vi "config serial port.vi"(8 "error in (no error)":errorcluster) -> (0 "error out":errorcluster, 3 "reference out":refnum<visa-resource-name>)   [LabVIEW 2020]
uses:
  Ardunio Type.ctl
  <vilib>/Instr/_visa.llb/VISA Find Search Mode.ctl
  <vilib>/Instr/_visa.llb/VISA Configure Serial Port (Instr).vi
panel:
  out "find list":string[](array[string])
  out "Array":string[](array[string])
  out "Arduino Found":bool
  in  "Arduino type":T1
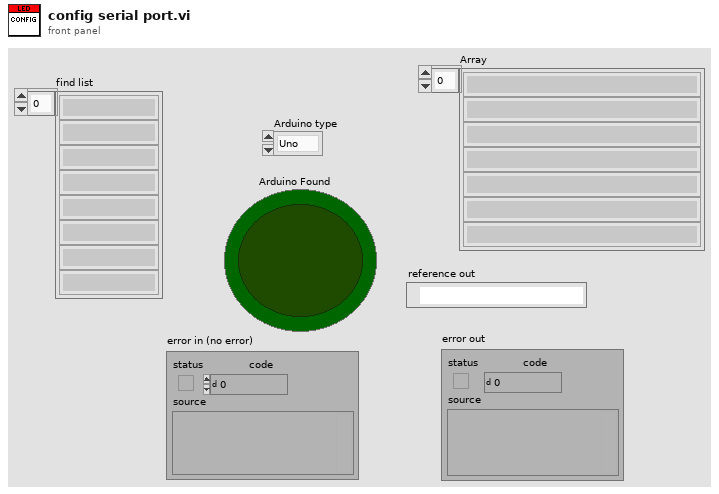
[diagram p1: front panel]
types:
  T1 = typedef "Ardunio Type.ctl" = enum16{"Uno", "Nano", "Micro"}
  T2 = typedef "VISA Find Search Mode.ctl" = u32
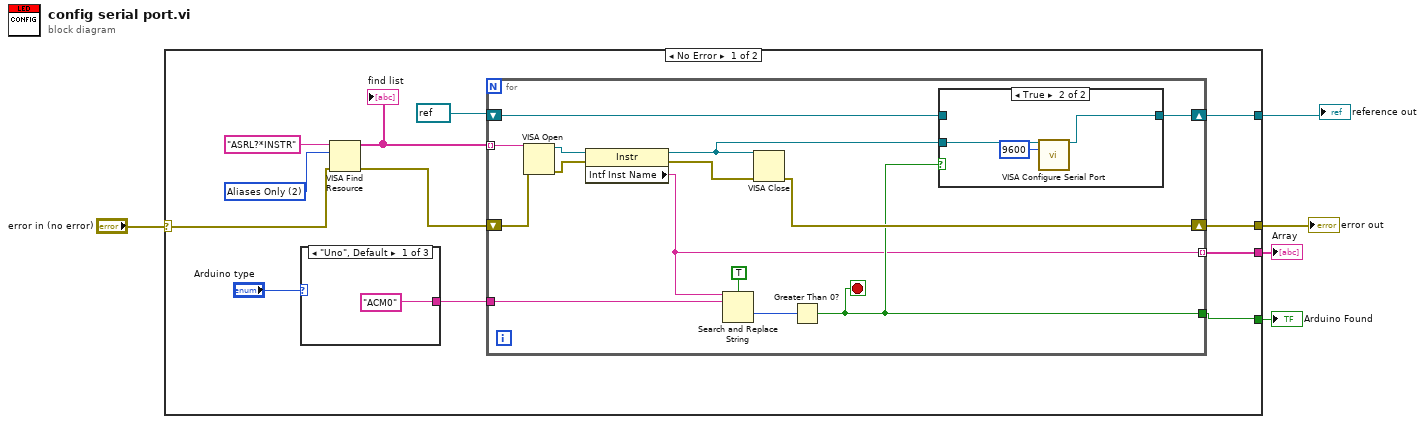
[diagram p0: block diagram]
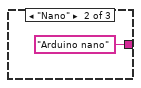
[diagram p2: hidden frame]
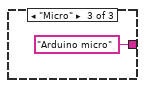
[diagram p3: hidden frame]
diagram:
  n1 = case shown="No Error" "error in (no error)" {
    selector: "error in (no error)" -> [w13 w39]
    tunnel: [w9 w39] -> w4
    tunnel: [w8 _] -> w3
    tunnel: [w7 _] -> w1
    tunnel: [w6 _] -> w2
    frame No Error {
      w16 = T2 2 items=["Canonical Names Only"=0, "Aliases Only"=2, "Include Matching Aliases"=3, "Include All Aliases"=4] ("Search Mode")
      n2 = case shown="\"Uno\", Default" "Arduino type" {
        tunnel: ["ACM0" ("search string") "Arduino nano" ("search string") "Arduino micro" ("search string")] -> w10
        frame "Uno", Default {
        }
        frame "Nano" {
        }
        frame "Micro" {
        }
      }
      n3 = VISA Find Resource(8:w13, 10:w16, 11:"ASRL?*INSTR" ("expression (\"?*\")")) -> (0:w14:errorcluster, 3:w15:string[])  [unwired: 1 out]
      "find list" <- w15
      n4 = for {
        tunnel: w15 -> [w34] mode=indexing
        shift-right: [w31] -> w8
        shift-left: refnum<visa-resource-name> refnum ("reference out") -> [w32]
        tunnel: w10 -> [w30]
        shift-right: [w25] -> w9
        shift-left: w14 -> [w26]
        tunnel: [w21] -> w7 mode=indexing
        tunnel: [w22] -> w6
        stop <- w22 stop-if-true
        n5 = VISA Open(error in (no error)=w26, VISA resource name=w34) -> (VISA resource name=w33:refnum<visa-resource-name>, error out=w27:errorcluster)  [unwired: 3 in]
        n6 = property class="Instr"(reference=w33, error in=w27) -> (reference out=w24:refnum<visa-resource-name>, error out=w28:errorcluster, "Intf Inst Name"=w21:string)
        n7 = Search and Replace String(case sensitive?=TRUE ("ignore case? (F)"), input string=w21, search string=w30) -> (offset past replacement=w23:i32)  [unwired: 5 in, 3 out]
        n8 = VISA Close(VISA resource name=w24, error in (no error)=w28) -> (error out=w25:errorcluster)
        n9 = Greater Than 0?(x=w23) -> (x > 0?=w22:bool)
        n10 = case shown="True" w22 {
          tunnel: w32 -> [w35 _]
          tunnel: [w35 w36] -> w31
          tunnel: w24 -> [_ w38]
          frame False {
          }
          frame True {
            n11 = call-poly "VISA Configure Serial Port"("VISA resource name"=w38, "baud rate (9600)"=u32 9600) -> ("VISA resource name out"=w36:refnum<visa-resource-name>)  [unwired: 12 in, 1 out]
          }
        }
      }
    }
    frame Error {
    }
  }
  "error out" <- w4
  "reference out" <- w3
  "Arduino Found" <- w2
  "Array" <- w1
